vi "Update eneble-disable measurement.vi"(8 "error in (no error)":errorcluster, 9 "MeasurementListBox":refnum<vi>, 10 "Current Position on Listbox":T1, 11 "Enabled?":bool=TRUE) -> (0 "error out":errorcluster)   [LabVIEW 2019, in "ZenGage v3.0 UI.lvclass"]
uses:
  ZenGage v3.0 UI.lvclass
  <vilib>/Utility/miscctls.llb/LVRowAndColumnTypeDef.ctl
  <vilib>/Utility/miscctls.llb/LVPoint32TypeDef.ctl
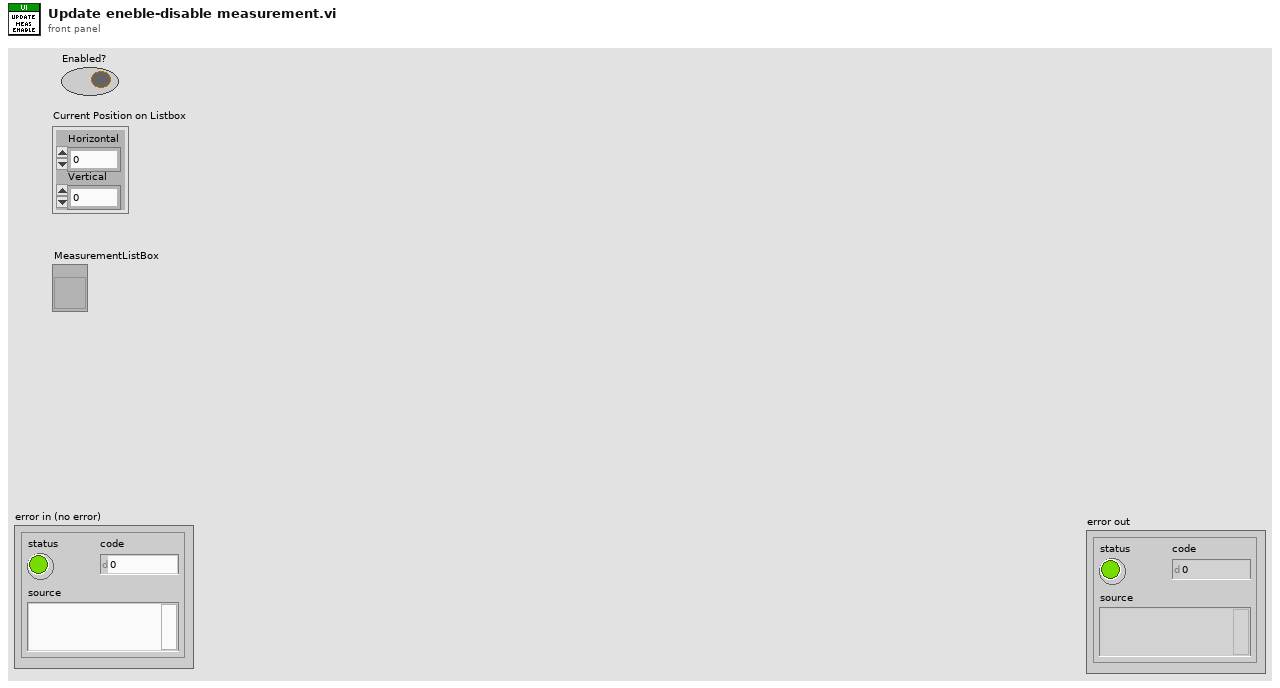
[diagram p1: front panel]
types:
  T1 = typedef "LVPoint32TypeDef.ctl" = cluster{"Horizontal":i32, "Vertical":i32}
  T2 = typedef "LVRowAndColumnTypeDef.ctl" = cluster{"Row":i32, "Column":i32}
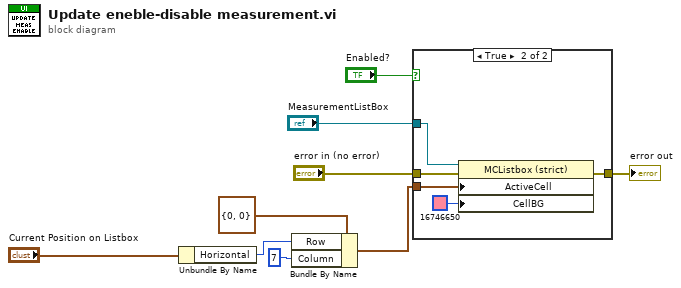
[diagram p0: block diagram]
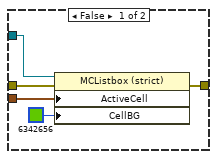
[diagram p2: hidden frame]
diagram:
  n1 = Unbundle By Name("Current Position on Listbox") -> ("Horizontal"=w7:i32)
  n2 = Bundle By Name(cluster=T2 {"Row"=0, "Column"=0} ("Active Cell:Active Cell"), "Row"=w7, "Column"=7) -> (w5:T2)
  n3 = case shown="True" "Enabled?" {
    tunnel: "MeasurementListBox" -> [w14 w18]
    tunnel: w5 -> [w13 w17]
    tunnel: "error in (no error)" -> [w11 w16]
    tunnel: [w10 w15] -> w2
    frame False {
      n4 = property class="MCListbox (strict)"(reference=w14, error in=w11, "ActiveCell"=w13, "CellBG"=u32 6342656) -> (error out=w10:errorcluster)  [unwired: 1 out]
    }
    frame True {
      n5 = property class="MCListbox (strict)"(reference=w18, error in=w16, "ActiveCell"=w17, "CellBG"=u32 16746650) -> (error out=w15:errorcluster)  [unwired: 1 out]
    }
  }
  "error out" <- w2
